vi "Initialize Async.vi"(6 "Parameters":T8[](array[typedef]) {"Base Word" format="%04d"}, 8 "error in (no error)":errorcluster, 10 "Async Message Config":T1={"Group"=0, "High Priority"=FALSE, "Time to Next Msg (100 us)"=0, "Command Config"={"Command Type"=enum."Transmit", "Terminal Address"=enum."0", "SubAddress"=enum."1", "Word Count\\Mode Code"=enum."1", "Command Data"=[]}, "Message Control"={"MC17 Time Sync"=FALSE, "Error Mask"=FALSE, "Service Request Mask"=FALSE, "Busy Mask"=FALSE, "SubSystem Flag Mask"=FALSE, "Terminal Flag Mask"=FALSE, "Reserved Mask"=FALSE, "Retry"=FALSE, "Bus A / !Bus B"=FALSE, "Self-Test Loopback"=FALSE, "Broadcast Mask"=FALSE, "EoM Interrupt"=FALSE, "Mode Code Format"=FALSE, "Broadcast Format"=FALSE, "RT-RT Format"=FALSE}} {"Group" format="%04x"}, 11 "ID":string) -> (0 "error out":errorcluster, 3 "Async Message out":refnum<class "Async Message.lvclass">)   [LabVIEW 2020, in "BCI-1553 API.lvlib" / "Async Message.lvclass"]
doc: "Generates an Asynchronous Message object that can be sent out on a Bus Controller subcomponent. The Async Message has all the same properties and requirements as a normal Message but may only be sent out after the Bus Controller has started. An Async Message can be high or low priority. High priority Messages get sent out as soon as there is time to do so in-between the execution of Messages. Low priority Messages are sent out between the execution of Minor Frames,if there is enough time to do so. The Group value should always be set to 0."
uses:
  Async Message.lvclass
  TypeDefs/Simplified Parameter Data Table.ctl
  TypeDefs/Scaling Information.ctl
  TypeDefs/Async Message Config.ctl
  TypeDefs/Command Config.ctl
  TypeDefs/Command Type.ctl
  TypeDefs/Command Terminal Address.ctl
  TypeDefs/Command SubAddress.ctl
  TypeDefs/Command Word Count.ctl
  TypeDefs/Message Control.ctl
  TypeDefs/Parameter Table Data.ctl
  Async Message.lvclass/Async Message.ctl
  BCI-1553 API.lvlib
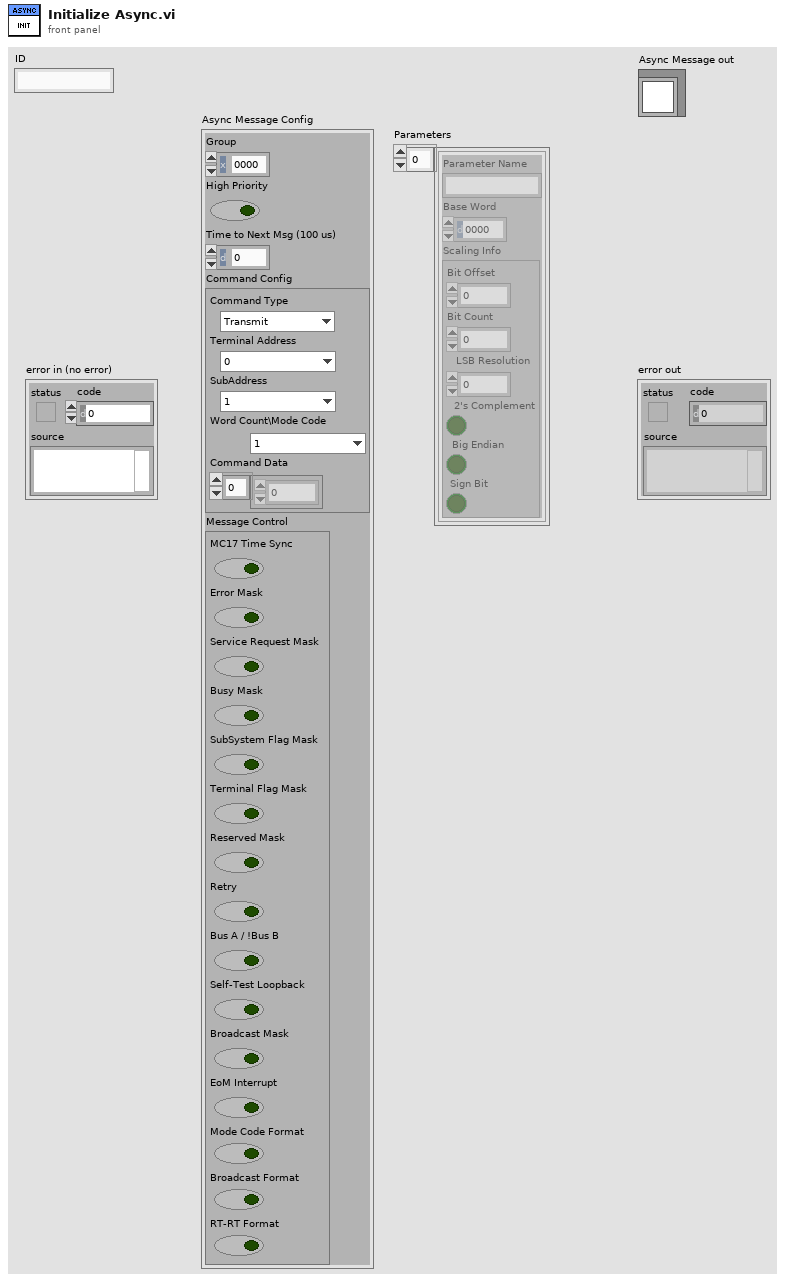
[diagram p1: front panel]
types:
  T1 = typedef "BCI-1553 API.lvlib/Async Message Config.ctl" = cluster{"Group":i32, "High Priority":bool, "Time to Next Msg (100 us)":u16, "Command Config":T2, "Message Control":T7}
  T2 = typedef "BCI-1553 API.lvlib/Command Config.ctl" = cluster{"Command Type":T3, "Terminal Address":T4, "SubAddress":T5, "Word Count\\Mode Code":T6, "Command Data":u16[]}
  T3 = typedef "BCI-1553 API.lvlib/Command Type.ctl" = enum16{"Transmit", "Receive"}
  T4 = typedef "BCI-1553 API.lvlib/Command Terminal Address.ctl" = enum16{"0", "1", "2", "3", "4", "5", "6", "7", "8", "9", "10", "11", "12", "13", "14", "15", "16", "17", "18", "19", "20", "21", "22", "23", "24", "25", "26", "27", "28", "29", "30", "Broadcast"}
  T5 = typedef "BCI-1553 API.lvlib/Command SubAddress.ctl" = enum16{"Mode Code", "1", "2", "3", "4", "5", "6", "7", "8", "9", "10", "11", "12", "13", "14", "15", "16", "17", "18", "19", "20", "21", "22", "23", "24", "25", "26", "27", "28", "29", "30"}
  T6 = typedef "BCI-1553 API.lvlib/Command Word Count.ctl" = enum16{"1", "2", "3", "4", "5", "6", "7", "8", "9", "10", "11", "12", "13", "14", "15", "16", "17", "18", "19", "20", "21", "22", "23", "24", "25", "26", "27", "28", "29", "30", "31", "32"}
  T7 = typedef "BCI-1553 API.lvlib/Message Control.ctl" = cluster{"MC17 Time Sync":bool, "Error Mask":bool, "Service Request Mask":bool, "Busy Mask":bool, "SubSystem Flag Mask":bool, "Terminal Flag Mask":bool, "Reserved Mask":bool, "Retry":bool, "Bus A / !Bus B":bool, "Self-Test Loopback":bool, "Broadcast Mask":bool, "EoM Interrupt":bool, "Mode Code Format":bool, "Broadcast Format":bool, "RT-RT Format":bool}
  T8 = typedef "BCI-1553 API.lvlib/Simplified Parameter Data Table.ctl" = cluster{"Parameter Name":string, "Base Word":u16, "Scaling Info":T9}
  T9 = typedef "BCI-1553 API.lvlib/Scaling Information.ctl" = cluster{"Bit Offset":i32, "Bit Count":i32, "LSB Resolution":dbl, "2's Complement":bool, "Big Endian":bool, "Sign Bit":bool}
  T10 = typedef "BCI-1553 API.lvlib/Parameter Table Data.ctl" = cluster{"Parameter Name":string, "Base Word":u16, "Address":u16, "Value":u64, "Mask":u16[], "Scaling Info":T9}
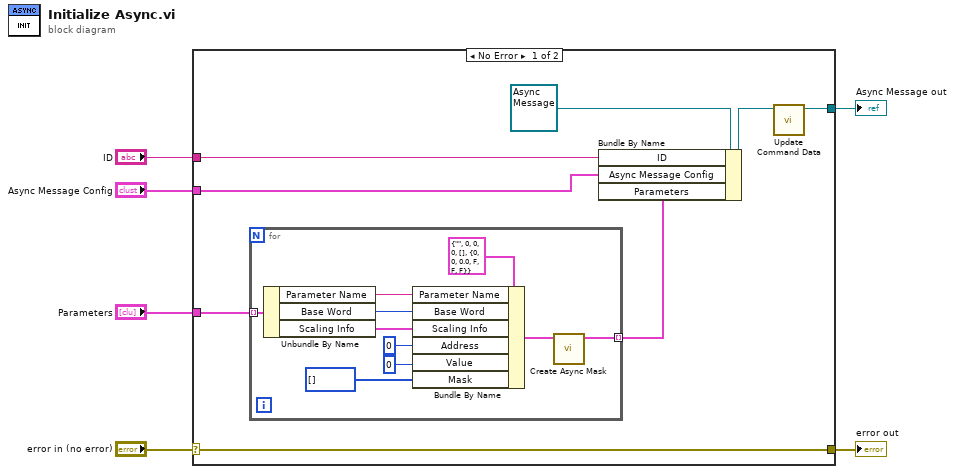
[diagram p0: block diagram]
diagram:
  n1 = case shown="No Error" "error in (no error)" {
    selector: "error in (no error)" -> [w14 w25]
    tunnel: [w14 w25] -> w5
    tunnel: [w9 _] -> w4
    tunnel: "ID" -> [w12 _]
    tunnel: "Parameters" -> [w7 _]
    tunnel: "Async Message Config" -> [w11 _]
    frame No Error {
      n2 = for {
        tunnel: w7 -> [w23] mode=indexing
        tunnel: [w15] -> w8 mode=indexing
        n3 = Unbundle By Name(w23) -> ("Parameter Name"=w22:string, "Base Word"=w21:u16, "Scaling Info"=w17:T9)
        n4 = Bundle By Name(cluster=T10 {"Parameter Name"="", "Base Word"=0, "Address"=0, "Value"=0, "Mask"=[], "Scaling Info"={"Bit Offset"=0, "Bit Count"=0, "LSB Resolution"=0.0, "2's Complement"=FALSE, "Big Endian"=FALSE, "Sign Bit"=FALSE}} ("Parameter Table Data"), "Parameter Name"=w22, "Base Word"=w21, "Scaling Info"=w17, "Address"=u16 0, "Value"=u64 0, "Mask"=u16[] []) -> (w16:T10)
        n5 = call "Create Async Mask.vi"("Parameter In"=w16) -> ("Parameter Out"=w15:T10)  [unwired: 9 in, 1 out]
      }
      n6 = Bundle By Name(cluster=refnum<class "Async Message.lvclass"> refnum ("Async Message in"), "ID"=w12, "Async Message Config"=w11, "Parameters"=w8) -> (w10:refnum<class "Async Message.lvclass">)
      n7 = call-dynamic "Update Command Data.vi"("Async Message in"=w10) -> ("Async Message out"=w9:refnum<class "Async Message.lvclass">)  [unwired: 9 in, 1 out]
    }
    frame Error {
    }
  }
  "error out" <- w5
  "Async Message out" <- w4
